vi "WL Pulse.vi"(8 "error in (no error)":errorcluster, 10 "Sample Rate":dbl=1000000.0, 11 "VWL (V)":dbl) -> (0 "error out":errorcluster)   [LabVIEW 2019]
uses:
  Globals.vi
  <vilib>/DAQmx/create/channels.llb/DAQmx Create Channel (AO-Voltage-Basic).vi
  <vilib>/DAQmx/configure/timing.llb/DAQmx Timing (Sample Clock).vi
  <vilib>/DAQmx/write.llb/DAQmx Write (Analog 1D Wfm NChan NSamp).vi
panel:
  out "AO Outputs":dbl[](array[numeric])
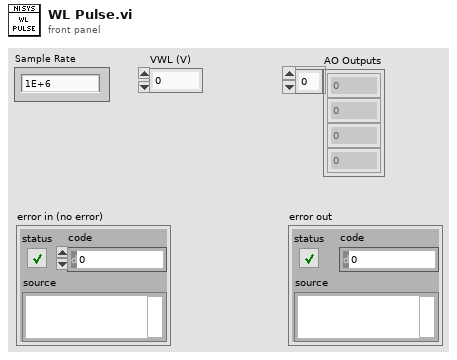
[diagram p1: front panel]
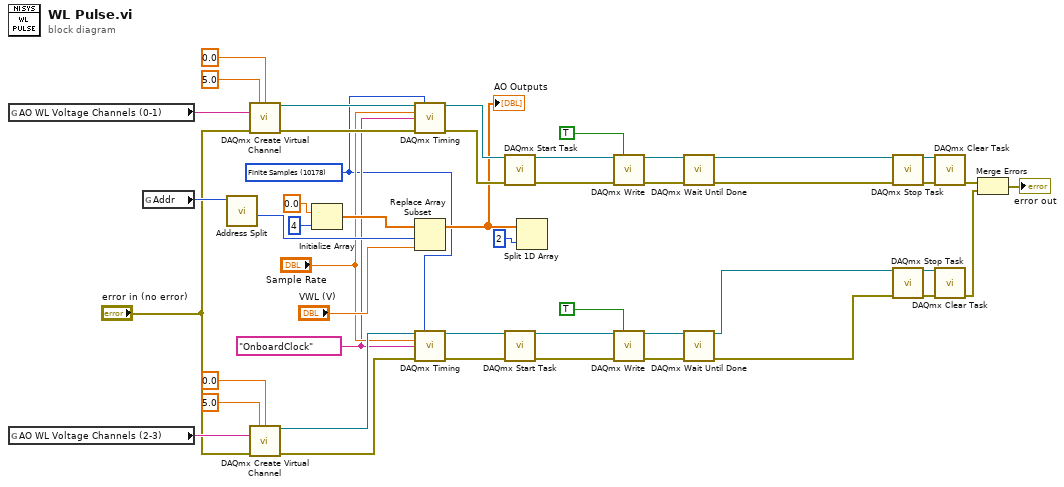
[diagram p0: block diagram]
diagram:
  w9 = 10178 items=["Finite Samples"=10178, "Continuous Samples"=10123, "Hardware Timed Single Point"=12522] ("sample mode")
  w14 = tag "OnboardClock" ("Sample Clock Source")
  n1 = global read "Globals.vi" "AO WL Voltage Channels (0-1)"() -> (w23:tag)
  n2 = global read "Globals.vi" "AO WL Voltage Channels (2-3)"() -> (w37:tag)
  n3 = global read "Globals.vi" "Addr"() -> (w43:u16)
  n4 = call "Address Split.vi"("address"=w43) -> ("wl_ext_sel"=w39:u32)  [unwired: 7 in, 3 out]
  n5 = call-poly <vilib>:"DAQmx Create Virtual Channel.vi"("maximum value"=5.0 ("Max Voltage"), "minimum value"=0.0 ("Min Voltage"), "physical channels"=w23, "error in"="error in (no error)") -> ("task out"=w13:refnum<k21>, "error out"=w22:errorcluster)  [unwired: 10 in]
  n6 = call-poly <vilib>:"DAQmx Create Virtual Channel.vi"("maximum value"=5.0 ("Max Voltage"), "minimum value"=0.0 ("Min Voltage"), "physical channels"=w37, "error in"="error in (no error)") -> ("task out"=w45:refnum<k21>, "error out"=w44:errorcluster)  [unwired: 10 in]
  n7 = Initialize Array(0.0 ("element"), 4 ("dimension size")) -> (w40:dbl[])
  n8 = call-poly <vilib>:"DAQmx Timing.vi"("task/channels in"=w13, "sample mode"=w9, "rate"="Sample Rate", "source"=w14, "error in"=w22) -> ("task out"=w24:refnum<k21>, "error out"=w25:errorcluster)  [unwired: 9 in]
  n9 = Replace Array Subset(array=w40, new element="VWL (V)", index=w39) -> (w12:dbl[])
  "AO Outputs" <- w12
  n10 = call-poly <vilib>:"DAQmx Timing.vi"("task/channels in"=w45, "sample mode"=w9, "rate"="Sample Rate", "source"=w14, "error in"=w44) -> ("task out"=w36:refnum<k21>, "error out"=w35:errorcluster)  [unwired: 9 in]
  n11 = call <vilib>:"DAQmx Start Task.vi"("task/channels in"=w24, "error in"=w25) -> ("task out"=w26:refnum<k21>, "error out"=w27:errorcluster)  [unwired: 12 in]
  n12 = call <vilib>:"DAQmx Start Task.vi"("task/channels in"=w36, "error in"=w35) -> ("task out"=w34:refnum<k21>, "error out"=w33:errorcluster)  [unwired: 12 in]
  n13 = Split 1D Array(array=w12, index=2) -> ()  [unwired: 2 out]
  n14 = call-poly <vilib>:"DAQmx Write.vi"("task/channels in"=w26, "auto start"=TRUE, "error in"=w27) -> ("task out"=w6:refnum<k21>, "error out"=w5:errorcluster)  [unwired: 10 in, 1 out]
  n15 = call-poly <vilib>:"DAQmx Write.vi"("task/channels in"=w34, "auto start"=TRUE, "error in"=w33) -> ("task out"=w8:refnum<k21>, "error out"=w7:errorcluster)  [unwired: 10 in, 1 out]
  n16 = call <vilib>:"DAQmx Wait Until Done.vi"("task/channels in"=w6, "error in"=w5) -> ("task out"=w4:refnum<k21>, "error out"=w3:errorcluster)  [unwired: 12 in]
  n17 = call <vilib>:"DAQmx Wait Until Done.vi"("task/channels in"=w8, "error in"=w7) -> ("task out"=w2:refnum<k21>, "error out"=w1:errorcluster)  [unwired: 12 in]
  n18 = call <vilib>:"DAQmx Stop Task.vi"("task/channels in"=w4, "error in"=w3) -> ("task out"=w29:refnum<k21>, "error out"=w28:errorcluster)  [unwired: 12 in]
  n19 = call <vilib>:"DAQmx Stop Task.vi"("task/channels in"=w2, "error in"=w1) -> ("task out"=w30:refnum<k21>, "error out"=w31:errorcluster)  [unwired: 12 in]
  n20 = call <vilib>:"DAQmx Clear Task.vi"("task in"=w29, "error in"=w28) -> ("error out"=w16:errorcluster)  [unwired: 13 in]
  n21 = call <vilib>:"DAQmx Clear Task.vi"("task in"=w30, "error in"=w31) -> ("error out"=w17:errorcluster)  [unwired: 13 in]
  n22 = Merge Errors(w16, w17) -> (→"error out":errorcluster)
